vi "AB_API Generate Error Cluster.vi"(8 "error in (no error)":errorcluster, 9 "error? (T)":bool=TRUE, 10 "Additional Message":string, 11 "Code":i32) -> (0 "error out":errorcluster={"status"=FALSE, "code"=0, "source"="\r\n"})   [LabVIEW 2020]
panel:
  in  "AB_API":string="AB_API"
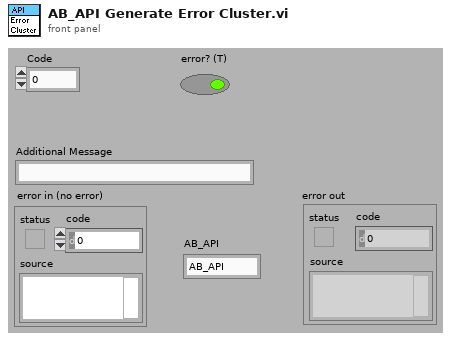
[diagram p1: front panel]
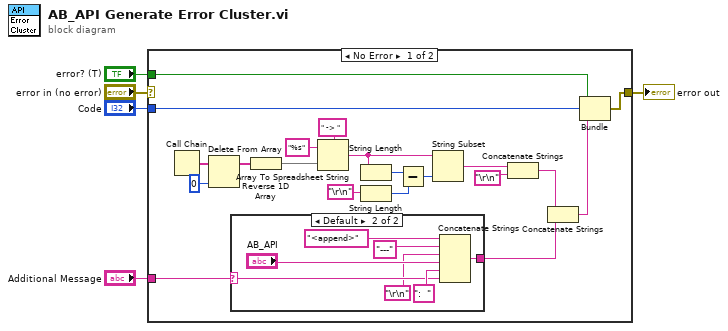
[diagram p0: block diagram]
diagram:
  n1 = case shown="No Error" "error in (no error)" {
    selector: "error in (no error)" -> [_ w34]
    tunnel: [w25 w34] -> w4
    tunnel: "Code" -> [w8 _]
    tunnel: "Additional Message" -> [w7 _]
    tunnel: "error? (T)" -> [w6 _]
    frame No Error {
      n2 = Call Chain() -> (call chain=w17:string[])
      n3 = Delete From Array(array=w17, index=0 ("Index")) -> (array with subset deleted=w12:string[])  [unwired: 1 in, 1 out]
      n4 = case shown="Default" w7 {
        selector: w7 -> [w26 w29]
        tunnel: [w26 w30] -> w21
        frame "" {
        }
        frame Default {
          n5 = Concatenate Strings("<append>", "---" ("string"), "\r\n", "AB_API", ":  " ("string"), w29) -> (w30:string)
        }
      }
      n6 = Reverse 1D Array(array=w12) -> (reversed array=w14:string[])
      n7 = Array To Spreadsheet String(delimiter (Tab)=" -> ", array=w14, 3:"%s" ("format string")) -> (spreadsheet string=w11:string)
      n8 = String Length(string=w11) -> (length=w15:i32)
      n9 = String Length(string="\r\n") -> (length=w9:i32)
      n10 = Subtract(x=w15, y=w9) -> (x-y=w16:i32)
      n11 = String Subset(string=w11, length (rest)=w16) -> (substring=w22:string)  [unwired: 1 in]
      n12 = Concatenate Strings(w22, "\r\n") -> (w23:string)
      n13 = Concatenate Strings(w23, w21) -> (w24:string)
      n14 = Bundle("error? (T)"=w6, "Code"=w8, w24) -> (w25:cluster{"error? (T)":bool, "Code":i32, string})  [unwired: 1 in]
    }
    frame Error {
      # "Cluster already contains error"
    }
  }
  "error out" <- w4
